vi "cm2nm_calc_trans_from_selected_session.vi"(0 "Current Session Information":T4, 9 "Sample_Information":T6 {"Session_list"."Instrument" items=["Unknown", "Phillips SEM IRC", "JEOL 7000F EML_MFC", "MXRD MFC", "JEOL_EPMA"]}, 11 "SessionIndex":i32=-1, 12 "TopLevelDataFilePath":path) -> (1 "CurrentRefSessionIdx":i32, 2 "CurrentSessionOut":T3[](array[typedef])=[{"MetaDataFile"=path "", "X"=-1.1, "Y"=0.0, "Z"=0.0, "Group"=0, "Rotation"=0.0, "Fiducial"=TRUE, "Magnification"=0.0, "Working_Distance"=0.0, "Notes"="", "Location Name/ID"="", "OtherRelatedDataFiles"=[], "Available"=FALSE}, {"MetaDataFile"=path "", "X"=0.0, "Y"=-1.0, "Z"=0.0, "Group"=0, "Rotation"=0.0, "Fiducial"=TRUE, "Magnification"=0.0, "Working_Distance"=0.0, "Notes"="", "Location Name/ID"="", "OtherRelatedDataFiles"=[], "Available"=FALSE}, {"MetaDataFile"=path "", "X"=0.0, "Y"=1.0, "Z"=0.0, "Group"=0, "Rotation"=0.0, "Fiducial"=TRUE, "Magnification"=0.0, "Working_Distance"=0.0, "Notes"="", "Location Name/ID"="", "OtherRelatedDataFiles"=[], "Available"=FALSE}, {"MetaDataFile"=path "", "X"=1.0, "Y"=0.0, "Z"=0.0, "Group"=0, "Rotation"=0.0, "Fiducial"=TRUE, "Magnification"=0.0, "Working_Distance"=0.0, "Notes"="", "Location Name/ID"="", "OtherRelatedDataFiles"=[], "Available"=FALSE}], 3 "ReferenceSession":T4={"CollectionOfPoints"=[{"MetaDataFile"=path "", "X"=50.1935, "Y"=19.379, "Z"=1.0, "Group"=0, "Rotation"=0.0, "Fiducial"=FALSE, "Magnification"=0.0, "Working_Distance"=0.0, "Notes"="", "Location Name/ID"="Interface_corrected", "OtherRelatedDataFiles"=[], "Available"=FALSE}, {"MetaDataFile"=path "", "X"=38.1101655, "Y"=26.3691263, "Z"=1.0, "Group"=0, "Rotation"=0.0, "Fiducial"=TRUE, "Magnification"=0.0, "Working_Distance"=0.0, "Notes"="", "Location Name/ID"="F1", "OtherRelatedDataFiles"=[], "Available"=TRUE}, {"MetaDataFile"=path "", "X"=43.2008536, "Y"=7.322264, "Z"=1.0, "Group"=0, "Rotation"=0.0, "Fiducial"=TRUE, "Magnification"=0.0, "Working_Distance"=0.0, "Notes"="", "Location Name/ID"="F3B", "OtherRelatedDataFiles"=[], "Available"=TRUE}, {"MetaDataFile"=path "", "X"=62.077256, "Y"=12.0875, "Z"=1.0, "Group"=0, "Rotation"=0.0, "Fiducial"=TRUE, "Magnification"=0.0, "Working_Distance"=0.0, "Notes"="", "Location Name/ID"="F5C", "OtherRelatedDataFiles"=[], "Available"=FALSE}, {"MetaDataFile"=path "", "X"=51.9658407, "Y"=19.1617677, "Z"=1.0, "Group"=0, "Rotation"=0.0, "Fiducial"=FALSE, "Magnification"=0.0, "Working_Distance"=0.0, "Notes"="", "Location Name/ID"="Corner_correcte_S1", "OtherRelatedDataFiles"=[], "Available"=FALSE}, {"MetaDataFile"=path "", "X"=51.947965, "Y"=19.1779565, "Z"=1.0, "Group"=0, "Rotation"=0.0, "Fiducial"=FALSE, "Magnification"=0.0, "Working_Distance"=0.0, "Notes"="", "Location Name/ID"="Corner_corrected_S2", "OtherRelatedDataFiles"=[], "Available"=FALSE}], "Instrument"=enum."JEOL 7000F EML_MFC", "CollectionFile"=path "/INL Macintosh/Users/timothymcjunkin/Desktop/Diffusion couple/JEOL 7000F SEM 9-3-10/Corrected_9-3-10.xlm", "Session Name/ID"="Correct_Abs_position", "SessionNotes"="EMSA images were taken off center so I May need to add the two together"}, 4 "PairedFiducialNames":T8(array[cluster]), 5 "FidcucialMetrics":cluster{"M1":dbl, "M2":dbl, "S1":dbl, "S2":dbl}, 6 "Matrices_in_text":string, 8 "Best_fit_and_name_match.":bool, 10 "transfrom_matrices":T1, 13 "NumberOfNameMatch":i32, 14 "OK_num_fids?":bool, 15 "ReferenceSession Name/ID":string)   [LabVIEW 2011]
doc: "Calculate the transformation to the current session from the selected previous session. \n\nThe routine selects the reference session sent in by the calling routine or if a negative number is sent as the value of SessionIndex the session just previous to the current session is used. The routine will decrement the session index if there are not at least three matching fiducials between the current session and the reference session. It will repeat this until it finds one or it arrives at the first session without a match.\n\nMatching is done by name. A check is made for the best fit algorithm and the flag Best_fit_and_name_match will be set if they are in agreement to the best match. This routine may is used as diagnostic in the future."
uses:
  cm2nm_sample_set.ctl
  cm2nm_coordinate_information_v2.ctl
  Instrument_type_enum_v2.ctl
  Sample_top_level.ctl
  Sample_Session_info.ctl
  transformMatrix.ctl
  <vilib>/Analysis/Matrix/Datatypes/RealMatrix.ctl
  <vilib>/Analysis/Matrix/NI_Matrix.lvlib
panel:
  out "Transform_from_theoretical":T1
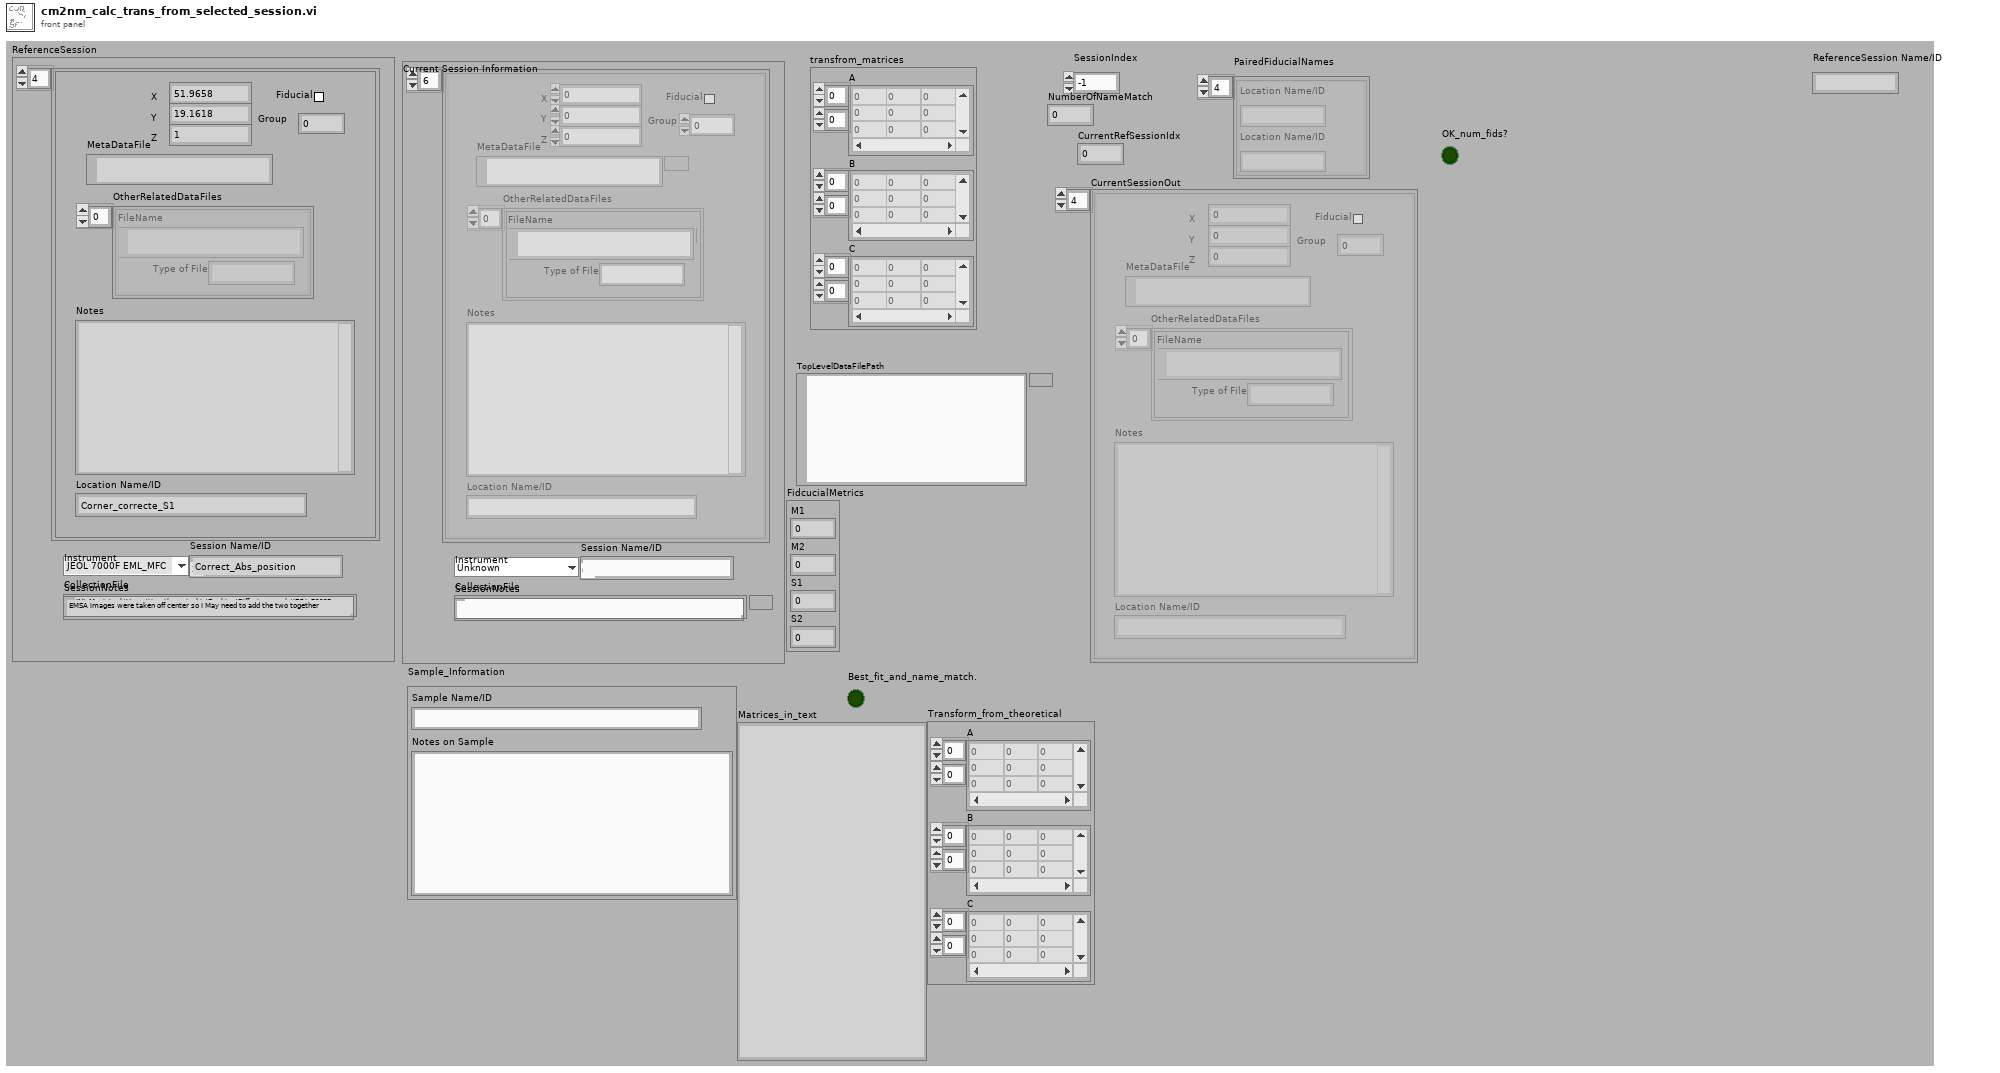
[diagram p1: front panel]
types:
  T1 = typedef "transformMatrix.ctl" = cluster{"A":T2, "B":T2, "C":T2}
  T2 = typedef "NI_Matrix.lvlib/RealMatrix.ctl" = dbl[][]
  T3 = typedef "cm2nm_coordinate_information_v2.ctl" = cluster{"MetaDataFile":path, "X":dbl, "Y":dbl, "Z":dbl, "Group":i32, "Rotation":dbl[unit], "Fiducial":bool, "Magnification":dbl, "Working_Distance":dbl, "Notes":string, "Location Name/ID":string, "OtherRelatedDataFiles":cluster{"Type of File":string, "FileName":path}[], "Available":bool}
  T4 = typedef "cm2nm_sample_set.ctl" = cluster{"CollectionOfPoints":T3[], "Instrument":T5, "CollectionFile":path, "Session Name/ID":string, "SessionNotes":string}
  T5 = typedef "Instrument_type_enum_v2.ctl" = enum16{"Unknown", "Philips FEI SEM IRC", "JEOL 7000F EML_MFC", "MXRD MFC", "JEOL_EPMA"}
  T6 = typedef "Sample_top_level.ctl" = cluster{"Sample Name/ID":string, "Notes on Sample":string, "Session_list":T7[]}
  T7 = typedef "Sample_Session_info.ctl" = cluster{"Instrument":u16, "Session_data_base":path, "Session Name/ID":string}
  T8 = cluster{"Location Name/ID":string, "Location Name/ID":string}[]
  T9 = cluster{"X1":dbl, "X2":dbl, "Y1":dbl, "Y2":dbl, "Z1":dbl, "Z2":dbl}[]
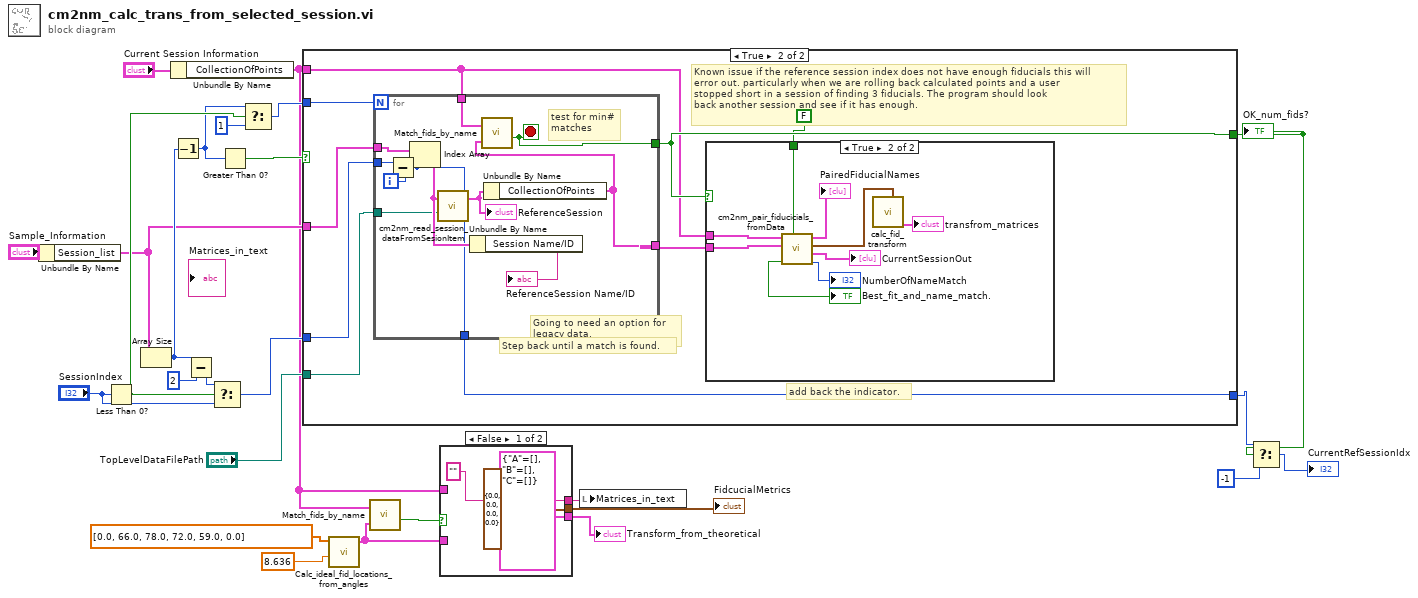
[diagram p0: block diagram]
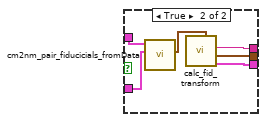
[diagram p2: hidden frame]
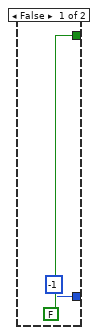
[diagram p3: hidden frame]
diagram:
  n1 = Unbundle By Name("Sample_Information") -> ("Session_list"=w17:T7[])
  n2 = Less Than 0?(x="SessionIndex") -> (x < 0?=w18:bool)
  n3 = Array Size(array=w17) -> (size(s)=w21:i32)
  n4 = Unbundle By Name("Current Session Information") -> ("CollectionOfPoints"=w6:T3[])
  n5 = Decrement(x=w21) -> (x-1=w14:i32)
  n6 = Subtract(x=w21, y=2) -> (x-y=w23:i32)
  n7 = Select(t=w23, s=w18, f="SessionIndex") -> (s? t:f=w16:i32)
  n8 = Greater Than 0?(x=w14) -> (x > 0?=w13:bool)
  n9 = Select(t=w14, s=w18, f=1) -> (s? t:f=w19:i32)
  n10 = case shown="True" w13 {
    tunnel: "TopLevelDataFilePath" -> [_ w37]
    tunnel: w19 -> [_ w36]
    tunnel: w17 -> [_ w35]
    tunnel: w16 -> [_ w34]
    tunnel: w6 -> [_ w29]
    tunnel: [FALSE ("AtLeast3") w32] -> w12
    tunnel: [-1 w30] -> w11
    frame False {
    }
    frame True {
      # "Going to need an option for\nlegacy data."
      # "Step back until a match is found."
      # "add back the indicator."
      # "Known issue if the reference session index does not have enough fiducials this will\nerror out. particularly when we are rolling back calculated points and a user\nstopped short in a session of finding 3 fiducials. The program should look\nback another session and see if it has enough."
      n11 = for {
        N: w36 -> [_]
        tunnel: w29 -> [w48]
        tunnel: w37 -> [w44]
        tunnel: w35 -> [w43]
        tunnel: w34 -> [w41]
        tunnel: [w40] -> w33
        tunnel: [w39] -> w32
        tunnel: [w38] -> w30
        i -> [w42]
        stop <- w39 stop-if-true
        # "test for min#\nmatches"
        n12 = Subtract(x=w41, y=w42) -> (x-y=w38:i32)
        n13 = Index Array(array=w43, index=w38) -> (element=w46:T7)
        n14 = call "cm2nm_read_session_dataFromSesionItem.vi"("TopLevelDataFilePath"=w44, "Sesions"=w46) -> ("Session_OUT"=w47:T4)  [unwired: 1 in]
        "ReferenceSession" <- w47
        n15 = Unbundle By Name(w46) -> ("Session Name/ID"=→"ReferenceSession Name/ID":string)
        n16 = Unbundle By Name(w47) -> ("CollectionOfPoints"=w40:T3[])
        n17 = call "Match_fids_by_name.vi"("CurrentSessionDataSet"=w48, "ReferenceSessionDataSet"=w40) -> ("AtLeast3"=w39:bool)  [unwired: 3 out]
      }
      n18 = case shown="True" w32 {
        tunnel: w29 -> [_ w54]
        tunnel: w33 -> [_ w53]
        tunnel: FALSE ("UseBestFit") -> [_ w51]
        frame False {
        }
        frame True {
          n19 = call "cm2nm_pair_fiducicials_fromData.vi"("CurrentSessionDataSet"=w54, "ReferenceSessionDataSet"=w53, "UseBestFit"=w51) -> ("CurrentSessionOut"=→"CurrentSessionOut":T3[], "Best_fit_and_name_match."=→"Best_fit_and_name_match.":bool, "PairedFiducialNames"=→"PairedFiducialNames":T8, "PairedFiducials"=w50:T9, "NumberOfNameMatch"=→"NumberOfNameMatch":i32)  [unwired: 3 out]
          n20 = call "calc_fid_transform.vi"("PairedFiducialCoordinates"=w50) -> ("Transformation_Matrices"=→"transfrom_matrices":T1)  [unwired: 2 in, 4 out]
        }
      }
    }
  }
  "OK_num_fids?" <- w12
  n21 = call "Calc_ideal_fid_locations_from_angles.vi"("r"=8.636 ("x"), "Array in"=dbl[] [0.0, 66.0, 78.0, 72.0, 59.0, 0.0]) -> ("Array out"=w3:T3[])  [unwired: 9 in]
  n22 = call "Match_fids_by_name.vi"("CurrentSessionDataSet"=w6, "ReferenceSessionDataSet"=w3) -> ("AtLeast3"=w7:bool)  [unwired: 3 out]
  n23 = case shown="False" w7 {
    tunnel: w6 -> [_ w66]
    tunnel: w3 -> [_ w65]
    tunnel: ["" ("Matrices_in_text") w63] -> w8
    tunnel: [T1 {"A"=[], "B"=[], "C"=[]} ("Transformation_Matrices") w62] -> w5
    tunnel: [cluster{"M1":dbl, "M2":dbl, "S1":dbl, "S2":dbl} {"M1"=0.0, "M2"=0.0, "S1"=0.0, "S2"=0.0} ("FidcucialMetrics") w61] -> w1
    frame False {
    }
    frame True {
      n24 = call "cm2nm_pair_fiducicials_fromData.vi"("CurrentSessionDataSet"=w66, "ReferenceSessionDataSet"=w65) -> ("PairedFiducials"=w64:T9)  [unwired: 1 in, 7 out]
      n25 = call "calc_fid_transform.vi"("PairedFiducialCoordinates"=w64) -> ("Transformation_Matrices"=w62:T1, "FidcucialMetrics"=w61:cluster{"M1":dbl, "M2":dbl, "S1":dbl, "S2":dbl}, "Matrices_in_text"=w63:string)  [unwired: 2 in, 2 out]
    }
  }
  "Transform_from_theoretical" <- w5
  "FidcucialMetrics" <- w1
  n26 = local write "Matrices_in_text"(w8) -> ()
  n27 = Select(t=w11, s=w12, f=-1) -> (s? t:f=→"CurrentRefSessionIdx":i32)
